vi "Value Change.vi"(7 "objects":T1, 8 "error in":errorcluster, 10 "EVENT":refnum<class "Abstract EVENT.lvclass">, 11 "Data Grid in":refnum<class "Data Grid.lvclass">) -> (0 "error out":errorcluster, 2 "Update?":bool, 3 "Data Grid out":refnum<class "Data Grid.lvclass">)   [LabVIEW 2013, in "Table Manager.lvlib" / "Data Grid.lvclass"]
uses:
  Data Grid.lvclass
  LabVIEWdotNetDataGrid/source/Events/Abstract EVENT/Abstract EVENT.lvclass
  TagSelectModule/Source/editor node/object ref.ctl
  <vilib>/NI/Tag Bus Data Framework/Configuration Editor/Classes/Engine Parent/Engine Parent Editor Node.lvclass
  <vilib>/NI/Tag Bus Data Framework/Configuration Editor/Classes/Module editor node/module editor node.lvclass
  <vilib>/NI/Tag Bus/tag/Data Type.ctl
  Table Manager/Cell Change.ctl
  Table Manager/Table Manager.lvclass/Table Manager.ctl
  Line/Line.lvclass/Line.ctl
  Column/Column.lvclass
  Column/Column.lvclass/Column.ctl
  Table Manager/Read Line.vi
  Line/Read Columns.vi
  TagSelectModule/Source/editor node/tag select module editor node.lvclass
  LabVIEWdotNetDataGrid/source/Events/CellValueChanged/CellValueChanged.lvclass
  Line/Line.lvclass
  Table Manager.lvlib
  <vilib>/NI/Tag Bus/tag/tag descriptor.lvclass
panel:
  in  "Enum":refnum<vi>
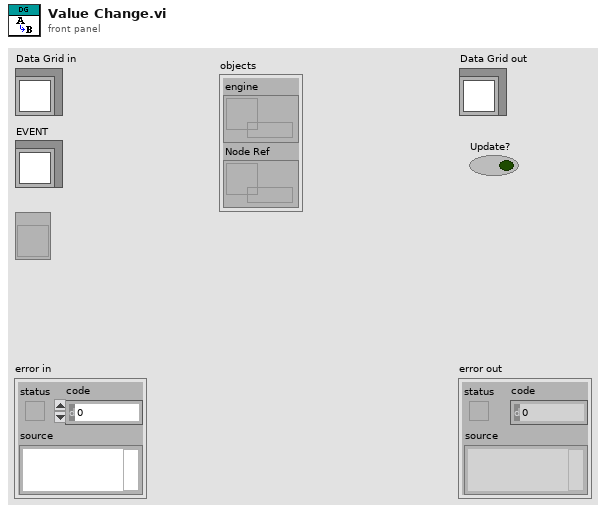
[diagram p1: front panel]
types:
  T1 = typedef "tag select module editor node.lvclass/object ref.ctl" = cluster{"engine":refnum<data-value>, "Node Ref":refnum<data-value>}
  T2 = typedef "Table Manager.lvlib/Cell Change.ctl" = cluster{"row":i32, "col":i32, "old name":string, "new name":string}
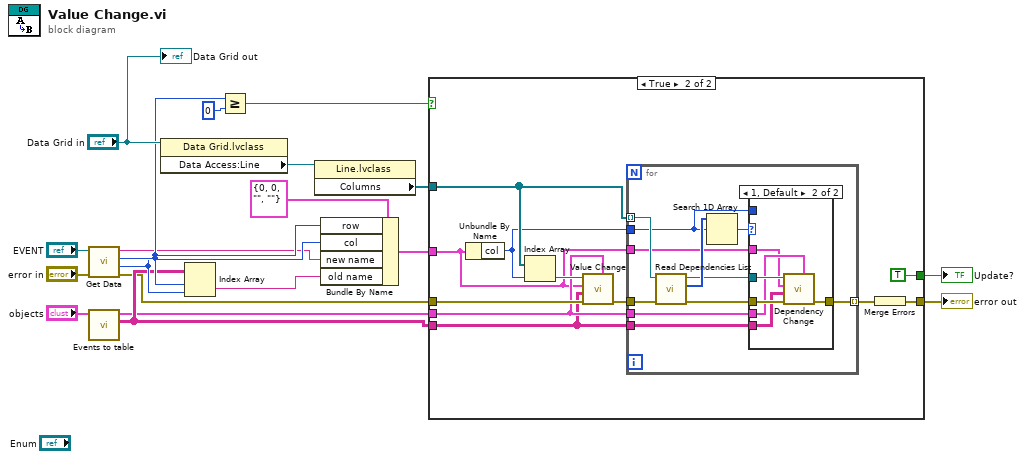
[diagram p0: block diagram]
diagram:
  n1 = call "Get Data.vi"("error in (no error)"="error in", "DataGrid.lvlib:Abstract EVENT.lvclass"="EVENT") -> ("error out"=w5:errorcluster, "column"=w9:i32, "row"=w10:i32, "cell value"=w8:string)  [unwired: 6 in]
  n2 = call "Events to table.vi"("object ref in"="objects") -> ("table"=w7:string[][], "object ref out"=w6:T1)  [unwired: 8 in, 1 out]
  n3 = property class="Data Grid.lvclass"(reference="Data Grid in") -> ("Data Access:Line"=w14:refnum<class "Line.lvclass">)  [unwired: 1 in, 2 out]
  n4 = Index Array(array=w7, index (row)=w10, index (col)=w9) -> (element=w1:string)
  n5 = Greater Or Equal?(x=w10, y=0) -> (x >= y?=w2:bool)
  n6 = property class="Line.lvclass"(reference=w14) -> ("Columns"=w13:refnum<class "Column.lvclass">[])  [unwired: 1 in, 2 out]
  n7 = Bundle By Name(cluster=T2 {"row"=0, "col"=0, "old name"="", "new name"=""} ("Cluster"), "row"=w10, "col"=w9, "new name"=w8, "old name"=w1) -> (w11:T2)
  n8 = case shown="True" w2 {
    tunnel: [w20 w29] -> w4
    tunnel: w13 -> [_ w27]
    tunnel: w5 -> [w20 w26]
    tunnel: w6 -> [_ w24]
    tunnel: w7 -> [_ w22]
    tunnel: w11 -> [_ w23]
    tunnel: [_ TRUE ("Update?")] -> w3
    frame False {
    }
    frame True {
      n9 = Unbundle By Name(w23) -> ("col"=w25:i32)
      n10 = Index Array(array=w27, index=w25) -> (element=w31:refnum<class "Column.lvclass">)
      n11 = call-dynamic "Value Change.vi"("object ref in"=w24, "error in (no error)"=w26, "old values"=w22, "Cluster"=w23, "Column in"=w31) -> ("error out"=w30:errorcluster)  [unwired: 5 in, 1 out]
      n12 = for {
        tunnel: w25 -> [w34]
        tunnel: w30 -> [w38]
        tunnel: [w42] -> w28 mode=indexing
        tunnel: w27 -> [w40] mode=indexing
        tunnel: w24 -> [w35]
        tunnel: w22 -> [w33]
        tunnel: w23 -> [w32]
        n13 = call "Read Dependencies List.vi"("error in (no error)"=w38, "Column in"=w40) -> ("error out"=w37:errorcluster, "Dependecies"=w41:i32[], "Column out"=w39:refnum<class "Column.lvclass">)  [unwired: 7 in]
        n14 = Search 1D Array(1D array=w41, element=w34) -> (index of element=w36:i32)  [unwired: 1 in]
        n15 = case shown="1, Default" w36 {
          tunnel: [w43 w49] -> w42
          tunnel: w37 -> [w43 w48]
          tunnel: w39 -> [_ w47]
          tunnel: w35 -> [_ w46]
          tunnel: w34 -> [_ _]
          tunnel: w33 -> [_ w45]
          tunnel: w32 -> [_ w44]
          frame -1 {
          }
          frame 1, Default {
            n16 = call-dynamic "Dependency Change.vi"("object ref in"=w46, "error in (no error)"=w48, "old values"=w45, "Cluster"=w44, "Column in"=w47) -> ("error out"=w49:errorcluster)  [unwired: 5 in, 1 out]
          }
        }
      }
      n17 = Merge Errors(w28) -> (w29:errorcluster)
    }
  }
  "error out" <- w4
  "Update?" <- w3
  "Data Grid out" <- "Data Grid in"
